vi "SV TDMS Read Octave (N Ch).vi"(0 "tdms file":refnum<k34>, 5 "group name in":string="Octave", 7 "channel names in":string[](array[string]), 11 "error in":errorcluster) -> (3 "scale labels":T1, 4 "tdms file out":refnum<k34>, 6 "group name out":string, 8 "channel names out":string[](array[string]), 10 "octave spectra":T2(array[cluster]), 13 "octave info":T3[](array[typedef]) {"engineering units" items=["custom..."=0, "V"=1, "A"=21, "C"=30, "pC"=31, "s"=32, "-"=29, "Pa"=2, "N"=20, "g"=3, "m/s^2"=4, "m/s"=5, "m"=6, "mm/s"=12, "mm"=13, "micron/s"=14, "micron"=15, "in/s^2"=7, "in/s"=8, "in"=9, "mil/s"=10, "mil"=11, "rad/s^2"=16, "rad/s"=17, "rad"=18, "deg/s^2"=26, "deg/s"=27, "deg"=28, "RPM"=22, "cycle/s^2"=23, "Hz"=24, "cycle"=25, "strain"=19]; "dB reference" format="%.2e"; "weighting filter" items=["Linear", "A-weighting", "B-weighting", "C-weighting", "ITU-R 468-4", "Dolby", "CCITT", "C-message", "Wb", "Wc", "Wd", "We", "Wf", "Wh", "Wj", "Wk", "Wm", "AES17 20 kHz lowpass", "AES17 40 kHz lowpass", "AES17 20 kHz highpass", "AES17 40 kHz highpass"]}, 15 "error out":errorcluster)   [LabVIEW 2017]
doc: "Reads the specified .tdms file and returns data in a format specific to the polymorphic instance selected."
uses:
  <vilib>/addons/_NISVFA/_Shared subVIs/Controls/svc_Octave Info.ctl
  <vilib>/addons/_NISVFA/_Shared subVIs/Controls/svc_Octave Standard.ctl
  <vilib>/addons/_NISVFA/_Shared subVIs/Controls/svc_Weighting Filter Text Ring.ctl
  <vilib>/addons/_NISVFA/_Shared subVIs/Controls/svc_Engineering Units Text Ring.ctl
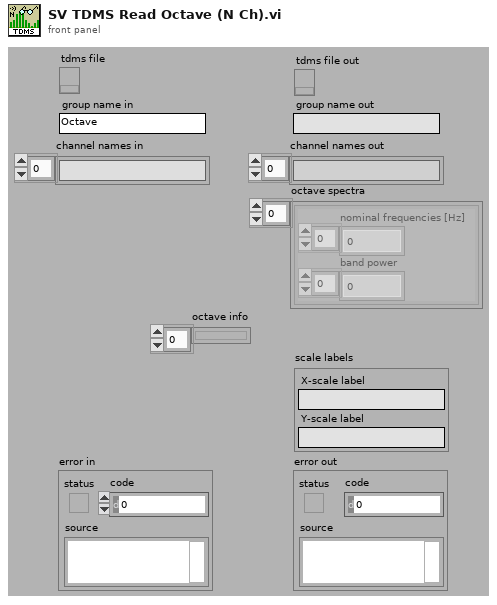
[diagram p1: front panel]
types:
  T1 = cluster{"X-scale label":string, "Y-scale label":string}
  T2 = cluster{"nominal frequencies [Hz]":dbl[], "band power":dbl[]}[]
  T3 = typedef "svc_Octave Info.ctl" = cluster{"standard":T4, "bandwidth":enum16{"1 octave", "1/3 octave", "1/6 octave", "1/12 octave", "1/24 octave"}, "low band":i32, "high band":i32, "weighting filter":T5, "dB reference":dbl, "dB On":bool, "unit label":string, "channel name":string, "description":string, "engineering units":T6, "custom label":string, "spectrum type":enum16{"power", "magnitude"}, "spectral density":bool, "filters settled":bool}
  T4 = typedef "svc_Octave Standard.ctl" = enum16{"ANSI S1.11", "IEC 61260"}
  T5 = typedef "svc_Weighting Filter Text Ring.ctl" = u16
  T6 = typedef "svc_Engineering Units Text Ring.ctl" = u16
  T7 = cluster{"nominal frequencies [Hz]":dbl[], "band power":dbl[]}
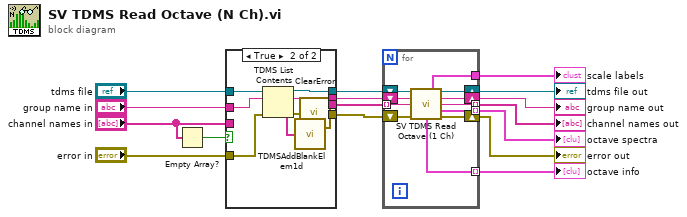
[diagram p0: block diagram]
diagram:
  n1 = Empty Array?(array="channel names in") -> (empty?=w16:bool)
  n2 = case shown="True" w16 {
    tunnel: [w19 w29] -> w15
    tunnel: [w18 w28] -> w8
    tunnel: [w20 w27] -> w9
    tunnel: [w17 w26] -> w10
    tunnel: "tdms file" -> [w19 w25]
    tunnel: "group name in" -> [w18 w24]
    tunnel: "channel names in" -> [w20 _]
    tunnel: "error in" -> [w17 w23]
    frame False {
    }
    frame True {
      n3 = TDMS List Contents(4:w23, 6:w24, 7:w25) -> (0:w21:errorcluster, 1:w22:string[], 2:w28:string, 3:w29:refnum<k34>)
      n4 = call <vilib>:"TDMSAddBlankElem1d.vi"("input string array"=w22) -> ("output string array with blank element at the beginning"=w27:string[])
      n5 = call <vilib>:"ClearError.vi"("error in (no error)"=w21) -> ("error out"=w26:errorcluster)
    }
  }
  n6 = for {
    shift-right: [w40] -> w14
    shift-left: w15 -> [w39]
    shift-right: [w37] -> w7
    shift-left: w8 -> [w38]
    tunnel: [w36] -> w6 mode=indexing
    shift-right: [w34] -> w4
    shift-left: w10 -> [w35]
    tunnel: [w33] -> w5 mode=indexing
    tunnel: [w32] -> w3 mode=indexing
    tunnel: w9 -> [w31] mode=indexing
    tunnel: [w30] -> w2
    n7 = call <vilib>:"SV TDMS Read Octave (1 Ch).vi"("tdms file"=w39, "group name in"=w38, "channel name in"=w31, "error in"=w35) -> ("scale labels"=w30:T1, "tdms file out"=w40:refnum<k34>, "group name out"=w37:string, "channel name out"=w36:string, "octave spectrum"=w33:T7, "octave info"=w32:T3, "error out"=w34:errorcluster)  [unwired: 5 in]
  }
  "error out" <- w4
  "tdms file out" <- w14
  "octave info" <- w3
  "octave spectra" <- w5
  "group name out" <- w7
  "channel names out" <- w6
  "scale labels" <- w2
